vi "Teleop.vi"(10 "Match Info":T1={"Autonomous Elapsed Seconds"=0.0, "TeleOp Elapsed Seconds"=0.0, "Disabled Elapsed Seconds"=0.0, "Visited Autonomous"=FALSE, "Visited TeleOp"=FALSE, "Visited Disabled"=FALSE, "Autonomous Settings"={"Autonomous Style"=enum."Independent", "VI Refnum"=refnum}}, 11 "Call Context":T2) -> ()   [LabVIEW 2016]
doc: "This VI is called for each enabled TeleOp packet received from the DS. It is typically used to read from joysticks and other inputs and update I/O or setpoints for timed control loops. It should complete and return within 20 milliseconds or risk missing DS packets."
uses:
  <vilib>/Rock Robotics/WPI/DriverStation/WPI_DriverStationDerivedRobotMode.ctl
  <vilib>/Rock Robotics/WPI/DriverStation/WPI_DriverStationMatch Info.ctl
  Support Code/Joystick Types.ctl
  <vilib>/Rock Robotics/WPI/Utilities/WPI_GetSetVariantRefNum.vi
  <vilib>/Rock Robotics/Network Tables/NT Write Boolean Array.vi
  <vilib>/Rock Robotics/Network Tables/NT Write Numeric Array.vi
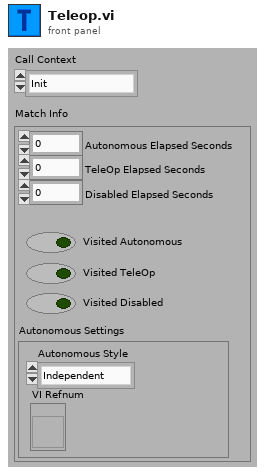
[diagram p1: front panel]
types:
  T1 = typedef "WPI_DriverStationMatch Info.ctl" = cluster{"Autonomous Elapsed Seconds":dbl, "TeleOp Elapsed Seconds":dbl, "Disabled Elapsed Seconds":dbl, "Visited Autonomous":bool, "Visited TeleOp":bool, "Visited Disabled":bool, "Autonomous Settings":cluster{"Autonomous Style":enum16{"Iterative", "Independent"}, "VI Refnum":refnum<vi>}}
  T2 = typedef "WPI_DriverStationDerivedRobotMode.ctl" = enum16{"Init", "Execute", "Stop"}
  T3 = typedef "Joystick Types.ctl" = enum16{"Extreme 3D Pro", "Xbox 360"}
  T4 = typedef "WPI_JoystickDevRef.ctl" = cluster{"Device":T5}
  T5 = typedef "WPI_JoystickDeviceEnum.ctl" = enum16{"USB 0", "USB 1", "USB 2", "USB 3", "USB 4", "USB 5"}
  T6 = cluster{"Buttons[0]":bool, "Buttons[1]":bool, "Buttons[2]":bool, "Buttons[3]":bool, "Buttons[4]":bool, "Buttons[5]":bool, "Buttons[6]":bool, "Buttons[7]":bool, "Buttons[8]":bool}
  T7 = typedef "CTRE_PigeonIMU_DeviceRef.ctl" = cluster{"DeviceStatus":errorcluster, "Device Number":u8, "Type":T8, "Device ID":u32}
  T8 = typedef "CTRE_PigeonIMU_ConnectionType.ctl" = u32
  T9 = typedef "CTRE_PigeonIMU_GlobalStatus.ctl" = cluster{"PigeonState":T10, "FusedHeading":cluster{"Heading":dbl, "Valid?":bool, "Fusing?":bool}, "YPR":cluster{"Yaw":dbl, "Pitch":dbl, "Roll":dbl}, "Compass":cluster{"Heading":dbl, "Magnitude":dbl, "Absolute Heading":dbl}, "Accelerometer":cluster{"Biased":cluster{"X":i16, "Y":i16, "Z":i16, "Norm":i16}, "Angles":cluster{"XZ Tilt":dbl, "YZ Tilt":dbl, "XY Tilt":dbl}}, "Magnetometer":cluster{"Raw":cluster{"X":i16, "Y":i16, "Z":i16}, "Biased":cluster{"X":i16, "Y":i16, "Z":i16}}, "Gyro":cluster{"X":dbl, "Y":dbl, "Z":dbl, "Norm":dbl}, "6D Quaternian":cluster{"W":dbl, "X":dbl, "Y":dbl, "Z":dbl}, "Temp. (C)":dbl, "UpTime":u32, "StartupStatus":cluster{"ResetCount":i32, "ResetFlags":i32, "FirmwareVersion":i32, "HasReset?":bool}, "Calibration":cluster{"CurrentMode":T11, "LastCalError":i32, "CalBooting?":bool}, "CAN Error":errorcluster, "AccumGyro":cluster{"X":dbl, "Y":dbl, "Z":dbl}, "Usage Frame":u32}
  T10 = typedef "CTRE_PigeonIMU_PigeonState.ctl" = enum16{"NoComm", "Initializing", "Ready", "UserCalibration"}
  T11 = typedef "CTRE_PigeonIMU_CalibrationMode.ctl" = u16
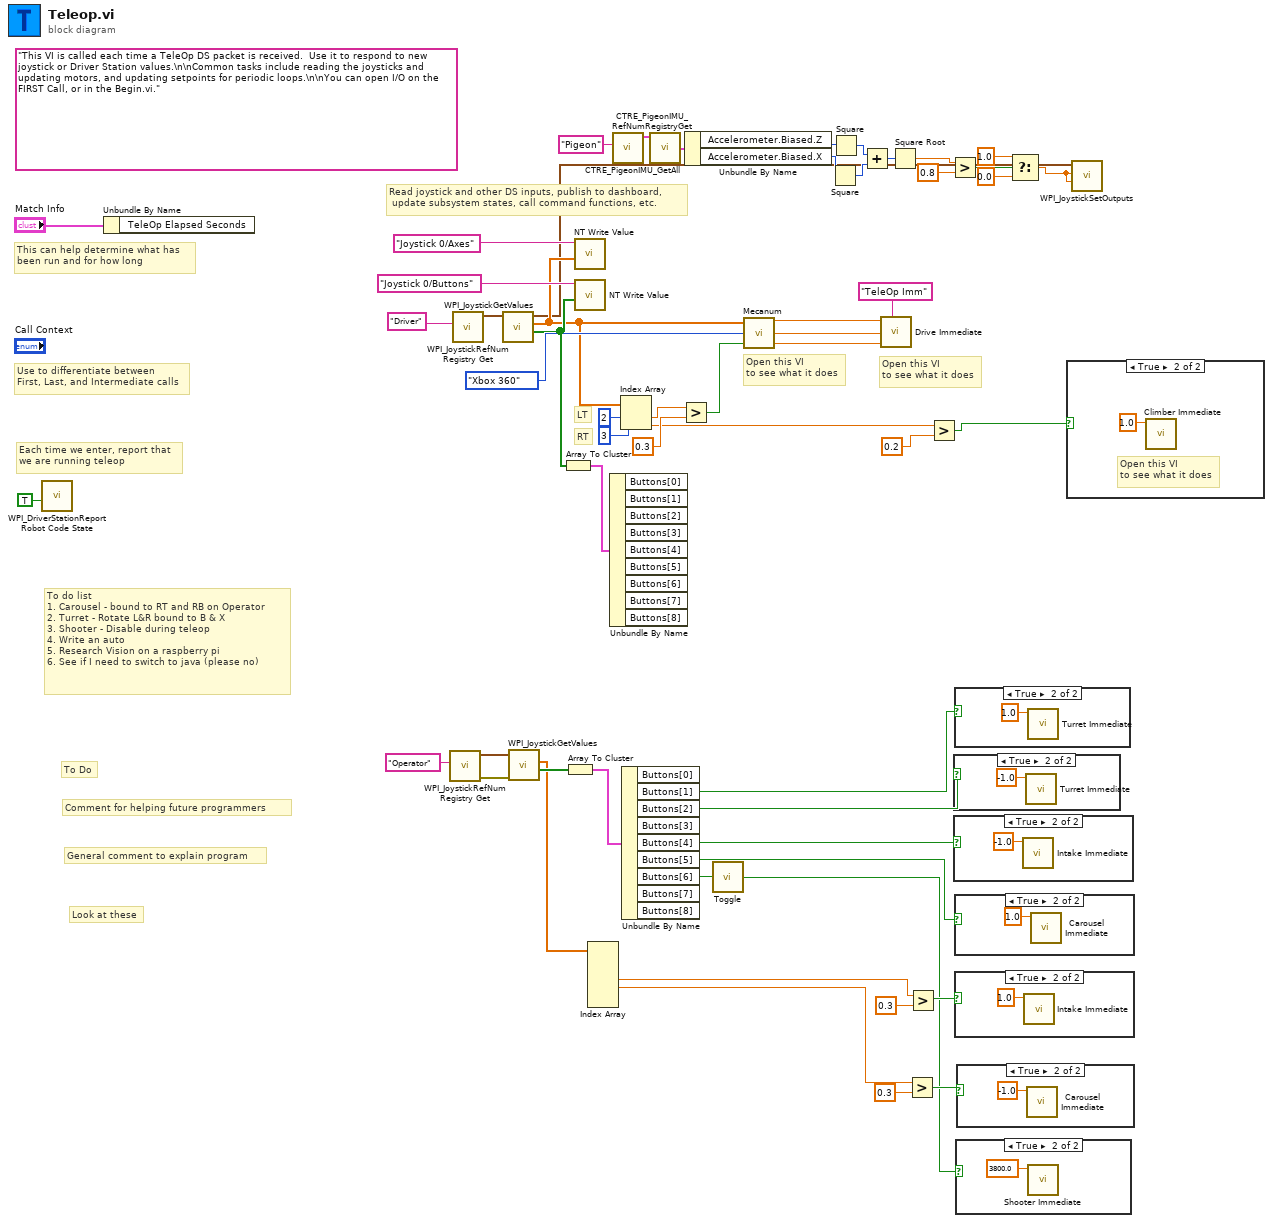
[diagram p0: block diagram]
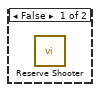
[diagram p2: hidden frame]
diagram:
  (unwired) "This VI is called each time a TeleOp DS packet is received.  Use it to respond to new joystick or Driver Station values.\n\nCommon tasks include reading the joysticks and updating motors, and updating setpoints for periodic loops.\n\nYou can open I/O on the FIRST Call, or in the Begin.vi."
  # "RT"
  # "LT"
  # "Open this VI\nto see what it does"
  # "Open this VI\nto see what it does"
  # "Look at these"
  # "General comment to explain program"
  # "Comment for helping future programmers"
  # "To Do"
  # "To do list\n1. Carousel - bound to RT and RB on Operator\n2. Turret - Rotate L&R bound to B & X\n3. Shooter - Disable during teleop\n4. Write an auto\n5. Research Vision on a raspberry pi\n6. See if I need to switch to java (please no)"
  # "Read joystick and other DS inputs, publish to dashboard,\n update subsystem states, call command functions, etc."
  # "Each time we enter, report that\nwe are running teleop"
  # "Use to differentiate between\nFirst, Last, and Intermediate calls"
  # "This can help determine what has\nbeen run and for how long"
  n1 = call <vilib>:"WPI_DriverStationReport Robot Code State.vi"("TeleOp"=TRUE ("Autonomous")) -> ()  [unwired: 10 in, 1 out]
  n2 = Unbundle By Name("Match Info") -> ()  [unwired: 1 out]
  n3 = call <vilib>:"WPI_JoystickRefNum Registry Get.vi"("refnum name"="Operator") -> ("error out"=w32:errorcluster, "JoystickDevRef"=w33:T4)  [unwired: 9 in]
  n4 = call <vilib>:"WPI_JoystickRefNum Registry Get.vi"("refnum name"="Driver") -> ("JoystickDevRef"=w52:T4)  [unwired: 1 in, 9 out]
  n5 = call <vilib>:"WPI_JoystickGetValues.vi"("JoystickDevRef"=w52) -> ("Buttons"=w46:bool[], "Axes"=w45:dbl[], "JoystickDevRef"=w10:T4)  [unwired: 6 in, 2 out]
  n6 = call <vilib>:"WPI_JoystickGetValues.vi"("error in (no error)"=w32, "JoystickDevRef"=w33) -> ("Buttons"=w30:bool[], "Axes"=w27:dbl[])  [unwired: 5 in, 3 out]
  n7 = Array To Cluster(array=w46) -> (cluster=w47:T6)
  n8 = Array To Cluster(array=w30) -> (cluster=w29:T6)
  n9 = call-poly <vilib>:"NT Write Value.vi"("Numeric Array"=w45, "Name"="Joystick 0/Axes") -> ()  [unwired: 9 in, 1 out]
  n10 = call-poly <vilib>:"NT Write Value.vi"("Boolean Array"=w46, "Name"="Joystick 0/Buttons") -> ()  [unwired: 9 in, 1 out]
  n11 = Index Array(array=w27) -> (element #3=w26:dbl, element #4=w5:dbl)  [unwired: 6 in, 4 out]
  n12 = Unbundle By Name(w47) -> ()  [unwired: 9 out]
  n13 = call <vilib>:"CTRE_PigeonIMU_RefNumRegistryGet.vi"("refnum name"="Pigeon") -> ("PigeonIMUDevRef"=w22:T7)  [unwired: 9 in, 1 out]
  n14 = Index Array(array=w45, index #1=2 ("index"), index #2=3 ("index")) -> (element #1=w42:dbl, element #2=w34:dbl)
  n15 = Unbundle By Name(w29) -> ("Buttons[1]"=w4:bool, "Buttons[2]"=w3:bool, "Buttons[4]"=w28:bool, "Buttons[5]"=w8:bool, "Buttons[6]"=w2:bool)  [unwired: 4 out]
  n16 = call <vilib>:"CTRE_PigeonIMU_GetAll.vi"("PigeonIMUDevRef"=w22) -> ("Get All"=w21:T9)  [unwired: 8 in, 2 out]
  n17 = Greater?(x=w42, y=0.3) -> (0:w41:bool)
  n18 = Unbundle By Name(w21) -> ("Accelerometer.Biased.Z"=w20:i16, "Accelerometer.Biased.X"=w19:i16)
  n19 = call "Toggle.vi"("Input"=w2) -> ("Output"=w1:bool)
  n20 = call "Mecanum.vi"("Low Speed Mode"=w41, "Controller Type"=Joystick_Types."Xbox 360", "Joystick Values"=w45) -> ("Spin"=w38:dbl, "Y Setpoint"=w39:dbl, "X Setpoint"=w40:dbl)
  n21 = Square(x=w19) -> (x^2=w18:i16)
  n22 = Square(x=w20) -> (x^2=w17:i16)
  n23 = Add(x=w17, y=w18) -> (x+y=w16:i16)
  n24 = call "Drive Immediate.vi"("Description"="TeleOp Imm", "Spin Setpoint"=w38, "Y Setpoint"=w39, "X Setpoint"=w40) -> ()  [unwired: 7 in, 1 out]
  n25 = Square Root(x=w16) -> (sqrt(x)=w15:dbl)
  n26 = Greater?(x=w5, y=0.3) -> (0:w7:bool)
  n27 = Greater?(x=w26, y=0.3) -> (0:w24:bool)
  n28 = Greater?(x=w34, y=0.2) -> (0:w36:bool)
  n29 = Greater?(x=w15, y=0.8) -> (0:w13:bool)
  n30 = case shown="True" w3 {
    frame False {
    }
    frame True {
      n31 = call "Turret Immediate.vi"("Setpoint"=-1.0) -> ()  [unwired: 10 in, 1 out]
    }
  }
  n32 = case shown="True" w28 {
    frame False {
    }
    frame True {
      n33 = call "Intake Immediate.vi"("Setpoint"=-1.0) -> ()  [unwired: 10 in, 1 out]
    }
  }
  n34 = case shown="True" w4 {
    frame False {
    }
    frame True {
      n35 = call "Turret Immediate.vi"("Setpoint"=1.0) -> ()  [unwired: 10 in, 1 out]
    }
  }
  n36 = case shown="True" w8 {
    frame False {
    }
    frame True {
      n37 = call "Carousel Immediate.vi"("Setpoint"=1.0) -> ()  [unwired: 10 in, 1 out]
    }
  }
  n38 = case shown="True" w24 {
    frame False {
    }
    frame True {
      n39 = call "Intake Immediate.vi"("Setpoint"=1.0) -> ()  [unwired: 10 in, 1 out]
    }
  }
  n40 = case shown="True" w1 {
    frame False {
      n41 = call "Reserve Shooter.vi"() -> ()  [unwired: 11 in, 1 out]
    }
    frame True {
      n42 = call "Shooter Immediate.vi"("Setpoint"=3800.0) -> ()  [unwired: 10 in, 1 out]
    }
  }
  n43 = case shown="True" w7 {
    frame False {
    }
    frame True {
      n44 = call "Carousel Immediate.vi"("Setpoint"=-1.0) -> ()  [unwired: 10 in, 1 out]
    }
  }
  n45 = Select(t=1.0, s=w13, f=0.0) -> (s? t:f=w9:dbl)
  n46 = case shown="True" w36 {
    frame False {
    }
    frame True {
      # "Open this VI\nto see what it does"
      n47 = call "Climber Immediate.vi"("Setpoint"=1.0) -> ()  [unwired: 10 in, 1 out]
    }
  }
  n48 = call <vilib>:"WPI_JoystickSetOutputs.vi"("Right Rumble"=w9, "Left Rumble"=w9, "JoystickDevRef"=w10) -> ()  [unwired: 7 in, 2 out]
